vi "GNC-2-1.vi"(11 "数组":u8[](array[numeric])) -> (1 "视速度增量":cluster{"X轴增量":i16, "Y轴增量":i16, "Z轴增量":i16}, 2 "角度增量":cluster{"X轴角增量":i16, "Y轴角增量":i16, "Z轴角增量":i16}, 3 "时间增量":i32)   [LabVIEW 2012]
uses:
  index-i16.vi
  XX-I16.vi
  index-i32.vi
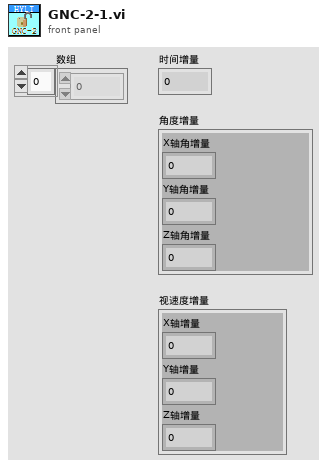
[diagram p1: front panel]
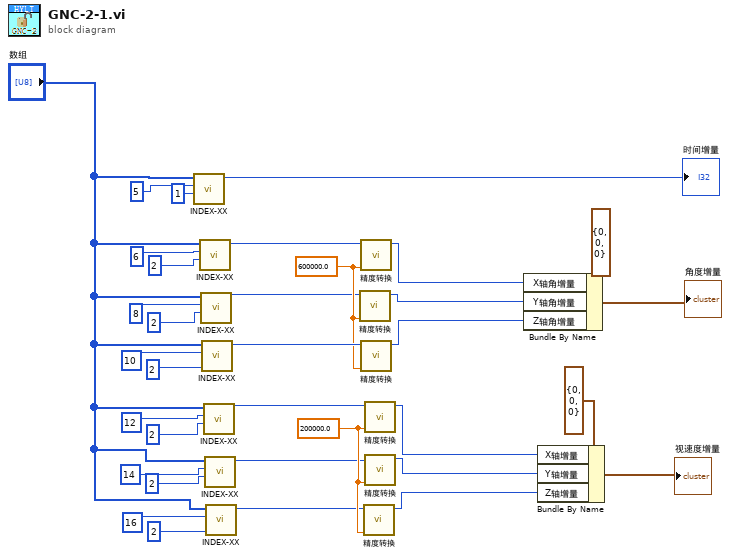
[diagram p0: block diagram]
diagram:
  w33 = 200000.0 ("单位")
  w24 = 600000.0 ("单位")
  n1 = call-poly "INDEX-XX.vi"("长度"=1, "索引"=5, "数组"="数组") -> ("数值输出"=→"时间增量":i32)  [unwired: 8 in]
  n2 = call-poly "INDEX-XX.vi"("长度"=2, "索引"=6, "数组"="数组") -> ("数值输出"=w20:i16)  [unwired: 8 in]
  n3 = call-poly "INDEX-XX.vi"("长度"=2, "索引"=8, "数组"="数组") -> ("数值输出"=w22:i16)  [unwired: 8 in]
  n4 = call-poly "INDEX-XX.vi"("长度"=2, "索引"=10, "数组"="数组") -> ("数值输出"=w25:i16)  [unwired: 8 in]
  n5 = call-poly "INDEX-XX.vi"("长度"=2, "索引"=12, "数组"="数组") -> ("数值输出"=w27:i16)  [unwired: 8 in]
  n6 = call-poly "INDEX-XX.vi"("长度"=2, "索引"=14, "数组"="数组") -> ("数值输出"=w29:i16)  [unwired: 8 in]
  n7 = call-poly "INDEX-XX.vi"("长度"=2, "索引"=16, "数组"="数组") -> ("数值输出"=w31:i16)  [unwired: 8 in]
  n8 = call-poly "精度转换.vi"("单位"=w24, "数值输入"=w22) -> ("输出"=w23:i16)  [unwired: 9 in]
  n9 = call-poly "精度转换.vi"("单位"=w24, "数值输入"=w20) -> ("输出"=w21:i16)  [unwired: 9 in]
  n10 = call-poly "精度转换.vi"("单位"=w24, "数值输入"=w25) -> ("输出"=w26:i16)  [unwired: 9 in]
  n11 = call-poly "精度转换.vi"("单位"=w33, "数值输入"=w31) -> ("输出"=w32:i16)  [unwired: 9 in]
  n12 = call-poly "精度转换.vi"("单位"=w33, "数值输入"=w27) -> ("输出"=w28:i16)  [unwired: 9 in]
  n13 = call-poly "精度转换.vi"("单位"=w33, "数值输入"=w29) -> ("输出"=w30:i16)  [unwired: 9 in]
  n14 = Bundle By Name(cluster=cluster{"X轴角增量":i16, "Y轴角增量":i16, "Z轴角增量":i16} {"X轴角增量"=0, "Y轴角增量"=0, "Z轴角增量"=0} ("角度增量"), "X轴角增量"=w21, "Y轴角增量"=w23, "Z轴角增量"=w26) -> (→"角度增量":cluster{"X轴角增量":i16, "Y轴角增量":i16, "Z轴角增量":i16})
  n15 = Bundle By Name(cluster=cluster{"X轴增量":i16, "Y轴增量":i16, "Z轴增量":i16} {"X轴增量"=0, "Y轴增量"=0, "Z轴增量"=0} ("视速度增量"), "X轴增量"=w28, "Y轴增量"=w30, "Z轴增量"=w32) -> (→"视速度增量":cluster{"X轴增量":i16, "Y轴增量":i16, "Z轴增量":i16})
